vi "TIO RPC Parse Reply Error.vi"(11 "Payload":string) -> (1 "Error Code":u16, 2 "Payload":string, 3 "Request ID":u16)   [LabVIEW 2016]
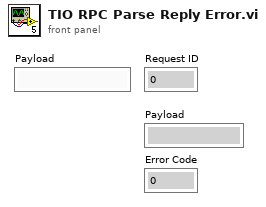
[diagram p1: front panel]
types:
  T1 = enum16{"big-endian, network order", "native, host order", "little-endian"}
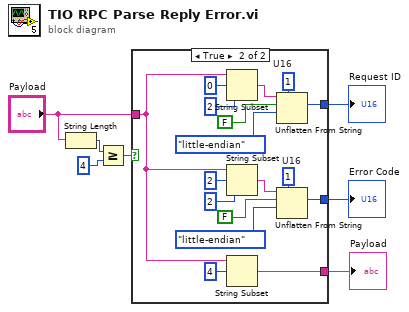
[diagram p0: block diagram]
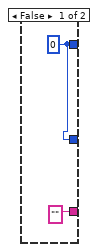
[diagram p2: hidden frame]
diagram:
  n1 = String Length(string="Payload") -> (length=w3:i32)
  n2 = Greater Or Equal?(x=w3, y=4) -> (x >= y?=w2:bool)
  n3 = case shown="True" w2 {
    tunnel: ["" ("Payload") w26] -> w7
    tunnel: [w8 w19] -> w6
    tunnel: "Payload" -> [_ w10]
    tunnel: [w8 w16] -> w1
    frame False {
      w8 = u16 0 ("U16")
    }
    frame True {
      w12 = u16 1  # U16
      w23 = u16 1  # U16
      n4 = String Subset(string=w10, offset (0)=0, length (rest)=2 ("length (rest)")) -> (substring=w20:string)
      n5 = String Subset(string=w10, offset (0)=2, length (rest)=2 ("length (rest)")) -> (substring=w15:string)
      n6 = String Subset(string=w10, offset (0)=4) -> (substring=w26:string)  [unwired: 1 in]
      n7 = Unflatten From String(type=w23, binary string=w20, data includes array or string size? (T)=FALSE, byte order (0:big-endian, network order)=T1."little-endian") -> (value=w19:u16)  [unwired: 1 in, 2 out]
      n8 = Unflatten From String(type=w12, binary string=w15, data includes array or string size? (T)=FALSE, byte order (0:big-endian, network order)=T1."little-endian") -> (value=w16:u16)  [unwired: 1 in, 2 out]
    }
  }
  "Payload" <- w7
  "Request ID" <- w6
  "Error Code" <- w1
